vi "Return Value Manifester VI Path.vi"(11 "Opaque Struct Writer in":refnum<class "Opaque Struct Writer.lvclass">) -> (2 "Manifester VI Path":path, 3 "Opaque Struct Writer out":refnum<class "Opaque Struct Writer.lvclass">)   [LabVIEW 2013, in "Opaque Struct Writer.lvclass"]
doc: "Copyright (c) 2016 Sze Howe Koh\n\nThis Source Code Form is subject to the terms of the Mozilla Public License, v. 2.0. If a copy of the MPL was not distributed with this file, You can obtain one at http://mozilla.org/MPL/2.0/."
uses:
  Opaque Struct Writer.lvclass
  Manifestation Writer/Manifestation Writer.lvclass/Manifestation Writer.ctl
  Manifestation Writer/Manifestation Writer.lvclass
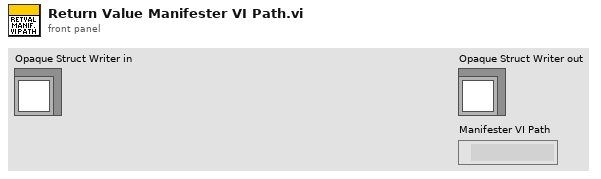
[diagram p1: front panel]
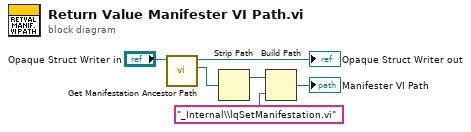
[diagram p0: block diagram]
diagram:
  n1 = call "Get Manifestation Ancestor Path.vi"("Manifestation Writer in"="Opaque Struct Writer in") -> ("Manifestation Ancestor Path"=w2:path, "Manifestation Writer out"=→"Opaque Struct Writer out":refnum<class "Opaque Struct Writer.lvclass">)  [unwired: 9 in]
  n2 = Strip Path(path=w2) -> (stripped path=w4:path)  [unwired: 1 out]
  n3 = Build Path(base path=w4, name or relative path="_Internal\\lqSetManifestation.vi") -> (appended path=→"Manifester VI Path":path)
